vi "Initial State Example - One-shot.vi"() -> ()   [LabVIEW 2018]
doc: "This example is meant to show the single-VI capability of the Initial State LabVIEW API. It works using a bucket you have already created in Initial State. It shows that once a bucket is created, you can stream to that bucket from anywhere in your system with this single VI. To use this example, you must have an Initial State account which can be created free at www.initialstate.com. You then create a bucket in Initial State, place the bucket key in the field along with your access key. Hit Run."
panel:
  out "Value":dbl format="%#_2g"
  in  "stop":bool
  in  "Stream Key":string="temperature"
  in  "error in (no error)":errorcluster
  in  "Bucket Key":string="FakeSHRkyOEAP"
  in  "Access Key":string="FakeFakeVj0GLMeSHRkyOEAPFGhzWEmw"
  # "This example is meant to work with a bucket already created in Initial State. It shows that once a bucket is created, you can stream to that bucket from anywhere in your system with this single VI. To use this example, create a bucket in Initial State, place the bucket key in the field along with your access key. Hit Run. NOTE: if you forget to create the bucket first, don't worry, you can still create a bucket with the same key and your data will be there."
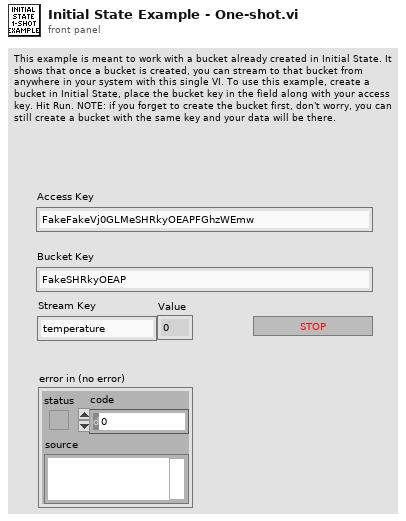
[diagram p1: front panel]
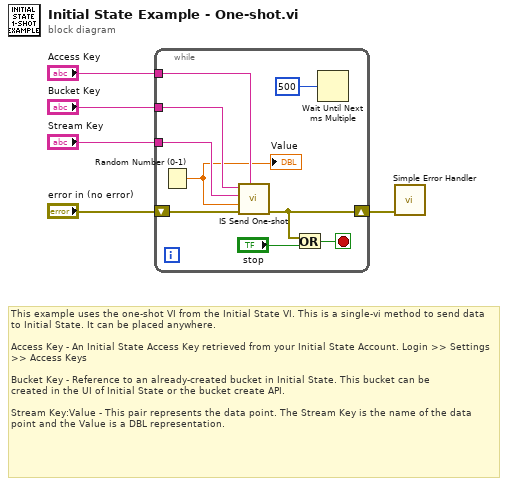
[diagram p0: block diagram]
diagram:
  # "This example uses the one-shot VI from the Initial State VI. This is a single-vi method to send data to Initial State. It can be placed anywhere. \n\nAccess Key - An Initial State Access Key retrieved from your Initial State Account. Login >> Settings >> Access Keys\n\nBucket Key - Reference to an already-created bucket in Initial State. This bucket can be \ncreated in the UI of Initial State or the bucket create API. \n\nStream Key:Value - This pair represents the data point. The Stream Key is the name of the data point and the Value is a DBL representation."
  n1 = while {
    tunnel: "Access Key" -> [w14]
    tunnel: "Bucket Key" -> [w12]
    tunnel: "Stream Key" -> [w11]
    shift-right: [w7] -> w1
    shift-left: "error in (no error)" -> [w13]
    stop <- w8 stop-if-true
    n2 = Random Number (0-1)() -> (number: 0 to 1=w10:dbl)
    "Value" <- w10
    n3 = call "IS Send One-shot.vi"("Access Key"=w14, "error in (no error)"=w13, "Numeric"=w10, "Stream Key"=w11, "Bucket Key"=w12) -> ("error out"=w7:errorcluster)  [unwired: 5 in, 1 out]
    n4 = Or(x=w7, y="stop") -> (x .or. y?=w8:bool)
    n5 = Wait Until Next ms Multiple(millisecond multiple=u32 500) -> ()  [unwired: 1 out]
  }
  n6 = call <vilib>:"Simple Error Handler.vi"("error in (no error)"=w1) -> ()  [unwired: 4 in, 5 out]
